vi "Build NT Ping Buffer.vi"() -> (3 "Data Buffer":string)   [LabVIEW 2017]
doc: "Build the ping message buffer for NT protocol."
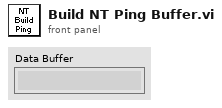
[diagram p1: front panel]
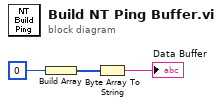
[diagram p0: block diagram]
diagram:
  n1 = Build Array(u8 0) -> (w2:u8[])
  n2 = Byte Array To String(unsigned byte array=w2) -> (string=→"Data Buffer":string)
